vi "GetEngineState.vi"(0 "Engine":refnum<class "Engine_1DO_2DI.lvclass">, 11 "error in (no error)":errorcluster) -> (4 "EngineState":T1=enum."Off", 6 "Automat":bool, 8 "Contactor":bool, 10 "DO Cmd":bool, 15 "error out":errorcluster)   [LabVIEW 2019, in "Engine_1DO_2DI.lvclass"]
uses:
  Engine_1DO_2DI.lvclass
  C:/Users/ANENKOV_V1/Desktop/src/Device_class/Device.lvclass
  TypeDef/State Engine.ctl
  Device_class/Device.lvclass/Device.ctl
  Engine_1DO_2DI.lvclass/Engine_1DO_2DI.ctl
  FPGA_API_class/FPGA API.lvclass
  Device_class/Device.lvclass
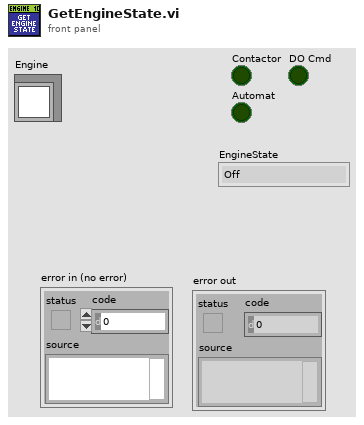
[diagram p1: front panel]
types:
  T1 = typedef "State Engine.ctl" = enum16{"Unknown", "Off", "TupningOn", "On", "TurningOff"}
  T2 = typedef "DI index.ctl" = u8
  T3 = typedef "DO index.ctl" = u8
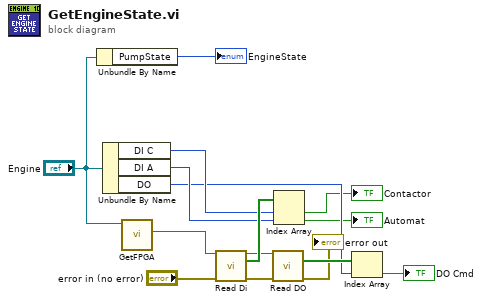
[diagram p0: block diagram]
diagram:
  n1 = Unbundle By Name("Engine") -> ("PumpState"=→"EngineState":T1)
  n2 = Unbundle By Name("Engine") -> ("DI C"=w13:T2, "DI A"=w12:T2, "DO"=w8:T3)
  n3 = call "GetFPGA.vi"("Device in"="Engine") -> ("FPGA API.lvclass"=w7:refnum<class "FPGA API.lvclass">)  [unwired: 10 in]
  n4 = call-dynamic "Read Di.vi"("FPGA API in"=w7, "error in (no error)"="error in (no error)") -> ("FPGA API out"=w10:refnum<class "FPGA API.lvclass">, "DIs"=w14:bool[], "error out"=w11:errorcluster)  [unwired: 11 in]
  n5 = call-dynamic "Read DO.vi"("FPGA API in"=w10, "error in (no error)"=w11) -> ("Ds"=w9:bool[], "error out"=→"error out":errorcluster)  [unwired: 11 in, 1 out]
  n6 = Index Array(array=w14, index #1=w13, index #2=w12) -> (element #1=→"Contactor":bool, element #2=→"Automat":bool)
  n7 = Index Array(array=w9, index=w8) -> (element=→"DO Cmd":bool)
